vi "Set Server State.vi"() -> ()   [LabVIEW 2009]
doc: "Use this interactiive VI to start and stop the XML-RPC server"
uses:
  Connection Parameters.ctl
panel:
  in  "Connection Parameters":T1={"address"="localhost", "remote port"=8080, "bytes to read"=10000, "read timeout ms (25000)"=25000, "write (request) timeout ms (25000)"=25000}
  in  "Update":bool
  in  "Server State":T2(ring)
  out "data out":string="HTTP/1.1 200 OK\nConnection: close\nContent-Length: 21400\nContent-Type: text/xml\nDate: Wed, 18 Apr 2007 08:18:48 GMT\nServer: LabVIEW 8.20/XP\n\n<?xml version=\"1.0\" encoding=\"UTF-8\"?>\n<methodResponse>\n  <params>\n    <param>\n      <array>\n  <data>\r<value><double>0.000000</double></value>\r<value><double>0.062791</double></value>\r<value><double>0.125333</double></value>\r<value><double>0.187381</double></value>\r<value><double>0.248690</double></value>\r<value><double>0.309017</double></value>\r<value><double>0.368125</double></value>\r<value><double>0.425779</double></value>\r<value><double>0.481754</double></value>\r<value><double>0.535827</double></value>\r<value><double>0.587785</double></value>\r<value><double>0.637424</double></value>\r<value><double>0.684547</double></value>\r<value><double>0.728969</double></value>\r<value><double>0.770513</double></value>\r<value><double>0.809017</double></value>\r<value><double>0.844328</double></value>\r<value><double>0.876307</double></value>\r<value><double>0.904827</double></value>\r<value><double>0.929776</double></value>\r<value><double>0.951057</double></value>\r<value><double>0.968583</double></value>\r<value><double>0.982287</double></value>\r<value><double>0.992115</double></value>\r<value><double>0.998027</double></value>\r<value><double>1.000000</double></value>\r<value><double>0.998027</double></value>\r<value><double>0.992115</double></value>\r<value><double>0.982287</double></value>\r<value><double>0.968583</double></value>\r<value><double>0.951057</double></value>\r<value><double>0.929776</double></value>\r<value><double>0.904827</double></value>\r<value><double>0.876307</double></value>\r<value><double>0.844328</double></value>\r<value><double>0.809017</double></value>\r<value><double>0.770513</double></value>\r<value><double>0.728969</double></value>\r<value><double>0.684547</double></value>\r<value><double>0.637424</double></value>\r<value><double>0.587785</double></value>\r<value><double>0.535827</double></value>\r<value><double>0.481754</double></value>\r<value><double>0.425779</double></value>\r<value><double>0.368125</double></value>\r<value><double>0.309017</double></value>\r<value><double>0.248690</double></value>\r<value><double>0.187381</double></value>\r<value><double>0.125333</double></value>\r<value><double>0.062791</double></value>\r<value><double>0.000000</double></value>\r<value><double>-0.062791</double></value>\r<value><double>-0.125333</double></value>\r<value><double>-0.187381</double></value>\r<value><double>-0.248690</double></value>\r<value><double>-0.309017</double></value>\r<value><double>-0.368125</double></value>\r<value><double>-0.425779</double></value>\r<value><double>-0.481754</double></value>\r<value><double>-0.535827</double></value>\r<value><double>-0.587785</double></value>\r<value><double>-0.637424</double></value>\r<value><double>-0.684547</double></value>\r<value><double>-0.728969</double></value>\r<value><double>-0.770513</double></value>\r<value><double>-0.809017</double></value>\r<value><double>-0.844328</double></value>\r<value><double>-0.876307</double></value>\r<value><double>-0.904827</double></value>\r<value><double>-0.929776</double></value>\r<value><double>-0.951057</double></value>\r<value><double>-0.968583</double></value>\r<value><double>-0.982287</double></value>\r<value><double>-0.992115</double></value>\r<value><double>-0.998027</double></value>\r<value><double>-1.000000</double></value>\r<value><double>-0.998027</double></value>\r<value><double>-0.992115</double></value>\r<value><double>-0.982287</double></value>\r<value><double>-0.968583</double></value>\r<value><double>-0.951057</double></value>\r<value><double>-0.929776</double></value>\r<value><double>-0.904827</double></value>\r<value><double>-0.876307</double></value>\r<value><double>-0.844328</double></value>\r<value><double>-0.809017</double></value>\r<value><double>-0.770513</double></value>\r<value><double>-0.728969</double></value>\r<value><double>-0.684547</double></value>\r<value><double>-0.637424</double></value>\r<value><double>-0.587785</double></value>\r<value><double>-0.535827</double></value>\r<value><double>-0.481754</double></value>\r<value><double>-0.425779</double></value>\r<value><double>-0.368125</double></value>\r<value><double>-0.309017</double></value>\r<value><double>-0.248690</double></value>\r<value><double>-0.187381</double></value>\r<value><double>-0.125333</double></value>\r<value><double>-0.062791</double></value>\r<value><double>0.000000</double></value>\r<value><double>0.062791</double></value>\r<value><double>0.125333</double></value>\r<value><double>0.187381</double></value>\r<value><double>0.248690</double></value>\r<value><double>0.309017</double></value>\r<value><double>0.368125</double></value>\r<value><double>0.425779</double></value>\r<value><double>0.481754</double></value>\r<value><double>0.535827</double></value>\r<value><double>0.587785</double></value>\r<value><double>0.637424</double></value>\r<value><double>0.684547</double></value>\r<value><double>0.728969</double></value>\r<value><double>0.770513</double></value>\r<value><double>0.809017</double></value>\r<value><double>0.844328</double></value>\r<value><double>0.876307</double></value>\r<value><double>0.904827</double></value>\r<value><double>0.929776</double></value>\r<value><double>0.951057</double></value>\r<value><double>0.968583</double></value>\r<value><double>0.982287</double></value>\r<value><double>0.992115</double></value>\r<value><double>0.998027</double></value>\r<value><double>1.000000</double></value>\r<value><double>0.998027</double></value>\r<value><double>0.992115</double></value>\r<value><double>0.982287</double></value>\r<value><double>0.968583</double></value>\r<value><double>0.951057</double></value>\r<value><double>0.929776</double></value>\r<value><double>0.904827</double></value>\r<value><double>0.876307</double></value>\r<value><double>0.844328</double></value>\r<value><double>0.809017</double></value>\r<value><double>0.770513</double></value>\r<value><double>0.728969</double></value>\r<value><double>0.684547</double></value>\r<value><double>0.637424</double></value>\r<value><double>0.587785</double></value>\r<value><double>0.535827</double></value>\r<value><double>0.481754</double></value>\r<value><double>0.425779</double></value>\r<value><double>0.368125</double></value>\r<value><double>0.309017</double></value>\r<value><double>0.248690</double></value>\r<value><double>0.187381</double></value>\r<value><double>0.125333</double></value>\r<value><double>0.062791</double></value>\r<value><double>0.000000</double></value>\r<value><double>-0.062791</double></value>\r<value><double>-0.125333</double></value>\r<value><double>-0.187381</double></value>\r<value><double>-0.248690</double></value>\r<value><double>-0.309017</double></value>\r<value><double>-0.368125</double></value>\r<value><double>-0.425779</double></value>\r<value><double>-0.481754</double></value>\r<value><double>-0.535827</double></value>\r<value><double>-0.587785</double></value>\r<value><double>-0.637424</double></value>\r<value><double>-0.684547</double></value>\r<value><double>-0.728969</double></value>\r<value><double>-0.770513</double></value>\r<value><double>-0.809017</double></value>\r<value><double>-0.844328</double></value>\r<value><double>-0.876307</double></value>\r<value><double>-0.904827</double></value>\r<value><double>-0.929776</double></value>\r<value><double>-0.951057</double></value>\r<value><double>-0.968583</double></value>\r<value><double>-0.982287</double></value>\r<value><double>-0.992115</double></value>\r<value><double>-0.998027</double></value>\r<value><double>-1.000000</double></value>\r<value><double>-0.998027</double></value>\r<value><double>-0.992115</double></value>\r<value><double>-0.982287</double></value>\r<value><double>-0.968583</double></value>\r<value><double>-0.951057</double></value>\r<value><double>-0.929776</double></value>\r<value><double>-0.904827</double></value>\r<value><double>-0.876307</double></value>\r<value><double>-0.844328</double></value>\r<value><double>-0.809017</double></value>\r<value><double>-0.770513</double></value>\r<value><double>-0.728969</double></value>\r<value><double>-0.684547</double></value>\r<value><double>-0.637424</double></value>\r<value><double>-0.587785</double></value>\r<value><double>-0.535827</double></value>\r<value><double>-0.481754</double></value>\r<value><double>-0.425779</double></value>\r<value><double>-0.368125</double></value>\r<value><double>-0.309017</double></value>\r<value><double>-0.248690</double></value>\r<value><double>-0.187381</double></value>\r<value><double>-0.125333</double></value>\r<value><double>-0.062791</double></value>\r<value><double>0.000000</double></value>\r<value><double>0.062791</double></value>\r<value><double>0.125333</double></value>\r<value><double>0.187381</double></value>\r<value><double>0.248690</double></value>\r<value><double>0.309017</double></value>\r<value><double>0.368125</double></value>\r<value><double>0.425779</double></value>\r<value><double>0.481754</double></value>\r<value><double>0.535827</double></value>\r<value><double>0.587785</double></value>\r<value><double>0.637424</double></value>\r<value><double>0.684547</double></value>\r<value><double>0.728969</double></value>\r<value><double>0.770513</double></value>\r<value><double>0.809017</double></value>\r<value><double>0.844328</double></value>\r<value><double>0.876307</double></value>\r<value><double>0.904827</double></value>\r<value><double>0.929776</double></value>\r<value><double>0.951057</double></value>\r<value><double>0.968583</double></value>\r<value><double>0.982287</double></value>\r<value><double>0.992115</double></value>\r<value><double>0.998027</double></value>\r<value><double>1.000000</double></value>\r<value><double>0.998027</double></value>\r<value><double>0.992115</double></value>\r<value><double>0.982287</double></value>\r<value><double>0.968583</double></value>\r<value><double>0.951057</double></value>\r<value><double>0.929776</double></value>\r<value><double>0.904827</double></value>\r<value><double>0.876307</double></value>\r<value><double>0.844328</double></value>\r<value><double>0.809017</double></value>\r<value><double>0.770513</double></value>\r<value><double>0.728969</double></value>\r<value><double>0.684547</double></value>\r<value><double>0.637424</double></value>\r<value><double>0.587785</double></value>\r<value><double>0.535827</double></value>\r<value><double>0.481754</double></value>\r<value><double>0.425779</double></value>\r<value><double>0.368125</double></value>\r<value><double>0.309017</double></value>\r<value><double>0.248690</double></value>\r<value><double>0.187381</double></value>\r<value><double>0.125333</double></value>\r<value><double>0.062791</double></value>\r<value><double>0.000000</double></value>\r<value><double>-0.062791</double></value>\r<value><double>-0.125333</double></value>\r<value><double>-0.187381</double></value>\r<value><double>-0.248690</double></value>\r<value><double>-0.309017</double></value>\r<value><double>-0.368125</double></value>\r<value><double>-0.425779</double></value>\r<value><double>-0.481754</double></value>\r<value><double>-0.535827</double></value>\r<value><double>-0.587785</double></value>\r<value><double>-0.637424</double></value>\r<value><double>-0.684547</double></value>\r<value><double>-0.728969</double></value>\r<value><double>-0.770513</double></value>\r<value><double>-0.809017</double></value>\r<value><double>-0.844328</double></value>\r<value><double>-0.876307</double></value>\r<value><double>-0.904827</double></value>\r<value><double>-0.929776</double></value>\r<value><double>-0.951057</double></value>\r<value><double>-0.968583</double></value>\r<value><double>-0.982287</double></value>\r<value><double>-0.992115</double></value>\r<value><double>-0.998027</double></value>\r<value><double>-1.000000</double></value>\r<value><double>-0.998027</double></value>\r<value><double>-0.992115</double></value>\r<value><double>-0.982287</double></value>\r<value><double>-0.968583</double></value>\r<value><double>-0.951057</double></value>\r<value><double>-0.929776</double></value>\r<value><double>-0.904827</double></value>\r<value><double>-0.876307</double></value>\r<value><double>-0.844328</double></value>\r<value><double>-0.809017</double></value>\r<value><double>-0.770513</double></value>\r<value><double>-0.728969</double></value>\r<value><double>-0.684547</double></value>\r<value><double>-0.637424</double></value>\r<value><double>-0.587785</double></value>\r<value><double>-0.535827</double></value>\r<value><double>-0.481754</double></value>\r<value><double>-0.425779</double></value>\r<value><double>-0.368125</double></value>\r<value><double>-0.309017</double></value>\r<value><double>-0.248690</double></value>\r<value><double>-0.187381</double></value>\r<value><double>-0.125333</double></value>\r<value><double>-0.062791</double></value>\r<value><double>0.000000</double></value>\r<value><double>0.062791</double></value>\r<value><double>0.125333</double></value>\r<value><double>0.187381</double></value>\r<value><double>0.248690</double></value>\r<value><double>0.309017</double></value>\r<value><double>0.368125</double></value>\r<value><double>0.425779</double></value>\r<value><double>0.481754</double></value>\r<value><double>0.535827</double></value>\r<value><double>0.587785</double></value>\r<value><double>0.637424</double></value>\r<value><double>0.684547</double></value>\r<value><double>0.728969</double></value>\r<value><double>0.770513</double></value>\r<value><double>0.809017</double></value>\r<value><double>0.844328</double></value>\r<value><double>0.876307</double></value>\r<value><double>0.904827</double></value>\r<value><double>0.929776</double></value>\r<value><double>0.951057</double></value>\r<value><double>0.968583</double></value>\r<value><double>0.982287</double></value>\r<value><double>0.992115</double></value>\r<value><double>0.998027</double></value>\r<value><double>1.000000</double></value>\r<value><double>0.998027</double></value>\r<value><double>0.992115</double></value>\r<value><double>0.982287</double></value>\r<value><double>0.968583</double></value>\r<value><double>0.951057</double></value>\r<value><double>0.929776</double></value>\r<value><double>0.904827</double></value>\r<value><double>0.876307</double></value>\r<value><double>0.844328</double></value>\r<value><double>0.809017</double></value>\r<value><double>0.770513</double></value>\r<value><double>0.728969</double></value>\r<value><double>0.684547</double></value>\r<value><double>0.637424</double></value>\r<value><double>0.587785</double></value>\r<value><double>0.535827</double></value>\r<value><double>0.481754</double></value>\r<value><double>0.425779</double></value>\r<value><double>0.368125</double></value>\r<value><double>0.309017</double></value>\r<value><double>0.248690</double></value>\r<value><double>0.187381</double></value>\r<value><double>0.125333</double></value>\r<value><double>0.062791</double></value>\r<value><double>0.000000</double></value>\r<value><double>-0.062791</double></value>\r<value><double>-0.125333</double></value>\r<value><double>-0.187381</double></value>\r<value><double>-0.248690</double></value>\r<value><double>-0.309017</double></value>\r<value><double>-0.368125</double></value>\r<value><double>-0.425779</double></value>\r<value><double>-0.481754</double></value>\r<value><double>-0.535827</double></value>\r<value><double>-0.587785</double></value>\r<value><double>-0.637424</double></value>\r<value><double>-0.684547</double></value>\r<value><double>-0.728969</double></value>\r<value><double>-0.770513</double></value>\r<value><double>-0.809017</double></value>\r<value><double>-0.844328</double></value>\r<value><double>-0.876307</double></value>\r<value><double>-0.904827</double></value>\r<value><double>-0.929776</double></value>\r<value><double>-0.951057</double></value>\r<value><double>-0.968583</double></value>\r<value><double>-0.982287</double></value>\r<value><double>-0.992115</double></value>\r<value><double>-0.998027</double></value>\r<value><double>-1.000000</double></value>\r<value><double>-0.998027</double></value>\r<value><double>-0.992115</double></value>\r<value><double>-0.982287</double></value>\r<value><double>-0.968583</double></value>\r<value><double>-0.951057</double></value>\r<value><double>-0.929776</double></value>\r<value><double>-0.904827</double></value>\r<value><double>-0.876307</double></value>\r<value><double>-0.844328</double></value>\r<value><double>-0.809017</double></value>\r<value><double>-0.770513</double></value>\r<value><double>-0.728969</double></value>\r<value><double>-0.684547</double></value>\r<value><double>-0.637424</double></value>\r<value><double>-0.587785</double></value>\r<value><double>-0.535827</double></value>\r<value><double>-0.481754</double></value>\r<value><double>-0.425779</double></value>\r<value><double>-0.368125</double></value>\r<value><double>-0.309017</double></value>\r<value><double>-0.248690</double></value>\r<value><double>-0.187381</double></value>\r<value><double>-0.125333</double></value>\r<value><double>-0.062791</double></value>\r<value><double>0.000000</double></value>\r<value><double>0.062791</double></value>\r<value><double>0.125333</double></value>\r<value><double>0.187381</double></value>\r<value><double>0.248690</double></value>\r<value><double>0.309017</double></value>\r<value><double>0.368125</double></value>\r<value><double>0.425779</double></value>\r<value><double>0.481754</double></value>\r<value><double>0.535827</double></value>\r<value><double>0.587785</double></value>\r<value><double>0.637424</double></value>\r<value><double>0.684547</double></value>\r<value><double>0.728969</double></value>\r<value><double>0.770513</double></value>\r<value><double>0.809017</double></value>\r<value><double>0.844328</double></value>\r<value><double>0.876307</double></value>\r<value><double>0.904827</double></value>\r<value><double>0.929776</double></value>\r<value><double>0.951057</double></value>\r<value><double>0.968583</double></value>\r<value><double>0.982287</double></value>\r<value><double>0.992115</double></value>\r<value><double>0.998027</double></value>\r<value><double>1.000000</double></value>\r<value><double>0.998027</double></value>\r<value><double>0.992115</double></value>\r<value><double>0.982287</double></value>\r<value><double>0.968583</double></value>\r<value><double>0.951057</double></value>\r<value><double>0.929776</double></value>\r<value><double>0.904827</double></value>\r<value><double>0.876307</double></value>\r<value><double>0.844328</double></value>\r<value><double>0.809017</double></value>\r<value><double>0.770513</double></value>\r<value><double>0.728969</double></value>\r<value><double>0.684547</double></value>\r<value><double>0.637424</double></value>\r<value><double>0.587785</double></value>\r<value><double>0.535827</double></value>\r<value><double>0.481754</double></value>\r<value><double>0.425779</double></value>\r<value><double>0.368125</double></value>\r<value><double>0.309017</double></value>\r<value><double>0.248690</double></value>\r<value><double>0.187381</double></value>\r<value><double>0.125333</double></value>\r<value><double>0.062791</double></value>\r<value><double>0.000000</double></value>\r<value><double>-0.062791</double></value>\r<value><double>-0.125333</double></value>\r<value><double>-0.187381</double></value>\r<value><double>-0.248690</double></value>\r<value><double>-0.309017</double></value>\r<value><double>-0.368125</double></value>\r<value><double>-0.425779</double></value>\r<value><double>-0.481754</double></value>\r<value><double>-0.535827</double></value>\r<value><double>-0.587785</double></value>\r<value><double>-0.637424</double></value>\r<value><double>-0.684547</double></value>\r<value><double>-0.728969</double></value>\r<value><double>-0.770513</double></value>\r<value><double>-0.809017</double></value>\r<value><double>-0.844328</double></value>\r<value><double>-0.876307</double></value>\r<value><double>-0.904827</double></value>\r<value><double>-0.929776</double></value>\r<value><double>-0.951057</double></value>\r<value><double>-0.968583</double></value>\r<value><double>-0.982287</double></value>\r<value><double>-0.992115</double></value>\r<value><double>-0.998027</double></value>\r<value><double>-1.000000</double></value>\r<value><double>-0.998027</double></value>\r<value><double>-0.992115</double></value>\r<value><double>-0.982287</double></value>\r<value><double>-0.968583</double></value>\r<value><double>-0.951057</double></value>\r<value><double>-0.929776</double></value>\r<value><double>-0.904827</double></value>\r<value><double>-0.876307</double></value>\r<value><double>-0.844328</double></value>\r<value><double>-0.809017</double></value>\r<value><double>-0.770513</double></value>\r<value><double>-0.728969</double></value>\r<value><double>-0.684547</double></value>\r<value><double>-0.637424</double></value>\r<value><double>-0.587785</double></value>\r<value><double>-0.535827</double></value>\r<value><double>-0.481754</double></value>\r<value><double>-0.425779</double></value>\r<value><double>-0.368125</double></value>\r<value><double>-0.309017</double></value>\r<value><double>-0.248690</double></value>\r<value><double>-0.187381</double></value>\r<value><double>-0.125333</double></value>\r<value><double>-0.062791</double></value>\r<value><double>0.000000</double></value>\r<value><double>0.062791</double></value>\r<value><double>0.125333</double></value>\r<value><double>0.187381</double></value>\r<value><double>0.248690</double></value>\r<value><double>0.309017</double></value>\r<value><double>0.368125</double></value>\r<value><double>0.425779</double></value>\r<value><double>0.481754</double></value>\r<value><double>0.535827</double></value>\r<value><double>0.587785</double></value>\r<value><double>0.637424</double></value>\n  </data>\n</array>\n    </param>\n  </params>\n</methodResponse>"
  out "call string":string="POST / HTTP/1.0\r\nContent-Type: text/xml\r\nUser-Agent: XML-RPC.NET\r\nHost: \r\nContent-Length: 315\n\n<?xml version=\"1.0\" encoding=\"UTF-8\"?>\n<methodCall>\n<methodName>Sine Wave.vi</methodName>\n  <params>\n<param>\n      <value><i4>512</i4></value>\n    </param><param>\n      <value><double>1.000000</double></value>\n    </param><param>\n      <value><double>0.010000</double></value>\n    </param>\n  </params>\n</methodCall>"
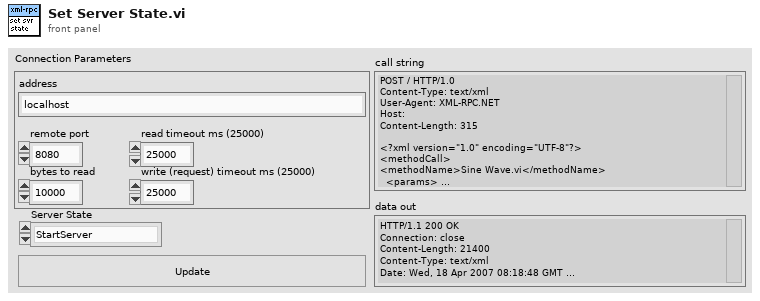
[diagram p1: front panel]
types:
  T1 = typedef "Connection Parameters.ctl" = cluster{"address":string, "remote port":u16, "bytes to read":i32, "read timeout ms (25000)":i32, "write (request) timeout ms (25000)":i32}
  T2 = enum16{"StartServer", "ShowServer", "HideServer", "EnableErrorLogging", "DisableErrorLogging", "StopServer"}
  T3 = enum32{"invalid app kind", "Development System", "Run Time System", "Student Edition", "Embedded LabVIEW", "Evaluation", "Custom"}
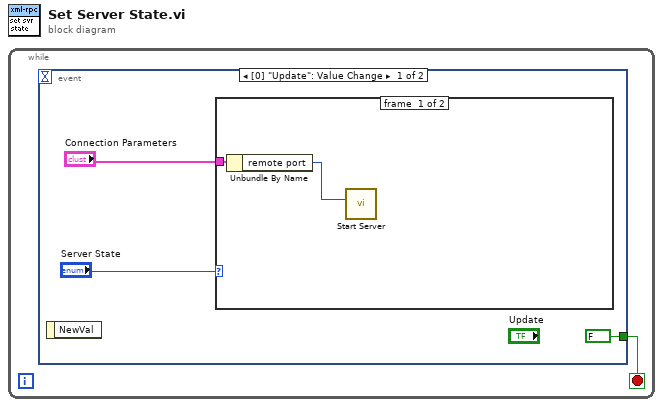
[diagram p0: block diagram]
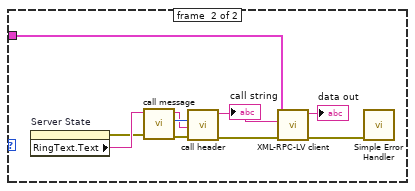
[diagram p2: hidden frame]
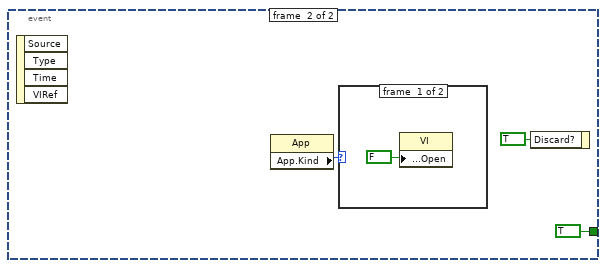
[diagram p3: hidden frame]
diagram:
  n1 = while {
    stop <- w1 stop-if-true
    n2 = event shown="[0] \"Update\": Value Change" {
      selector: _ -> [_ _]
      dyn-events: _ -> [_ _]
      timeout: _ -> [_ _]
      tunnel: [FALSE ("Update") TRUE ("Update")] -> w1
      event #0 {
        n3 = event-data() -> ()  [unwired: 1 in, 1 out]
        n4 = case shown="\"StartServer\"" "Server State" {
          tunnel: "Connection Parameters" -> [w6 w7]
          frame #0 {
            n5 = Unbundle By Name(w6) -> ("remote port"=w5:u16)
            n6 = call "Start Server.vi"("remote port"=w5) -> ()  [unwired: 11 in]
          }
          frame #1 {
            n7 = property on="Server State" class="Enum (strict)"() -> (error out=w9:errorcluster, "RingText.Text"=w10:string)  [unwired: 2 in, 1 out]
            n8 = call "call message.vi"("error in"=w9, "method name"=w10) -> ("error out"=w14:errorcluster, "length"=w16:i32, "response"=w15:string)  [unwired: 7 in]
            n9 = call "call header.vi"("error in"=w14, "Content String"=w15, "Content-Length"=w16) -> ("error out"=w12:errorcluster, "call string"=w13:string)  [unwired: 7 in]
            "call string" <- w13
            n10 = call "XML-RPC-LV client.vi"("error in (no error)"=w12, "method call"=w13, "Connection Parameters"=w7) -> ("error out"=w8:errorcluster, "method response"=→"data out":string)  [unwired: 7 in]
            n11 = call <vilib>:"Simple Error Handler.vi"("error in (no error)"=w8) -> ()  [unwired: 4 in, 5 out]
          }
        }
      }
      event #1 {
        n12 = event-data() -> ()  [unwired: 1 in, 4 out]
        n13 = property class="App"() -> ("App.Kind"=w17:T3)  [unwired: 2 in, 2 out]
        n14 = case shown="Default" w17 {
          frame #0 {
            n15 = property class="VI"("Front Panel.Open"=FALSE ("Front Panel Window:Open")) -> ()  [unwired: 2 in, 2 out]
          }
          frame #1 {
          }
        }
        n16 = event-data("Discard?"=TRUE) -> ()  [unwired: 1 in, 1 out]
      }
    }
  }
